vi "Read TrayStatus.vi"(8 "error in (no error)":errorcluster, 10 "F1/T2":bool, 11 "NG Pick in":refnum<class "NG Pick.lvclass">) -> (0 "error out":errorcluster, 1 "Arr_TrayST":bool[][](array[boolean]), 2 "Arr_Tray":cluster{"X":sgl, "Y":sgl}[][](array[cluster]), 3 "NG Pick out":refnum<class "NG Pick.lvclass">)   [LabVIEW 2019, in "NG Pick.lvclass"]
uses:
  NG Pick.lvclass
  Function/TraySet Folder/global/Tray_ArrAndData.vi
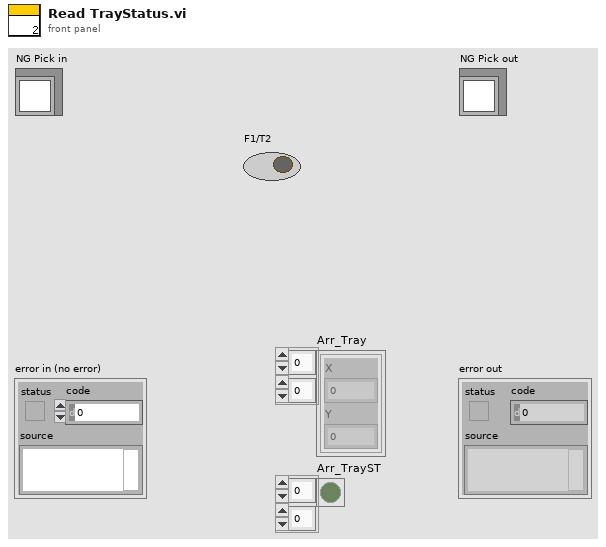
[diagram p1: front panel]
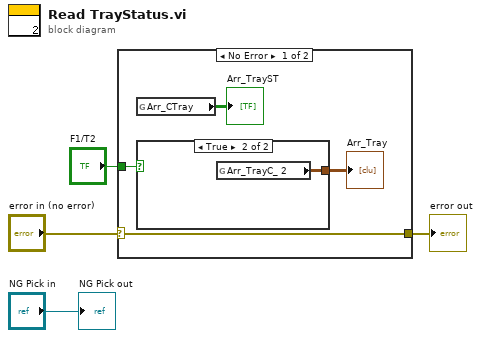
[diagram p0: block diagram]
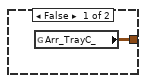
[diagram p2: hidden frame]
diagram:
  n1 = case shown="No Error" "error in (no error)" {
    selector: "error in (no error)" -> [w5 w11]
    tunnel: "F1/T2" -> [w7 _]
    tunnel: [w5 w11] -> w1
    frame No Error {
      n2 = global read "Tray_ArrAndData.vi" "Arr_CTray"() -> (→"Arr_TrayST":bool[][])
      n3 = case shown="True" w7 {
        tunnel: [w9 w10] -> w6
        frame False {
          n4 = global read "Tray_ArrAndData.vi" "Arr_TrayC_"() -> (w9:cluster{"X":sgl, "Y":sgl}[][])
        }
        frame True {
          n5 = global read "Tray_ArrAndData.vi" "Arr_TrayC_ 2"() -> (w10:cluster{"X":sgl, "Y":sgl}[][])
        }
      }
      "Arr_Tray" <- w6
    }
    frame Error {
    }
  }
  "error out" <- w1
  "NG Pick out" <- "NG Pick in"
